vi "Read (Digital Waveform).vi"(8 "error in (no error)":errorcluster, 9 "Timeout (10000 ms)":u32=10000, 11 "VISA resource name":refnum<visa-resource-name>) -> (0 "error out":errorcluster, 2 "Digital Waveform Graph":digitalwaveform(graph), 3 "VISA resource name out":refnum<visa-resource-name>)   [LabVIEW 2023, in "RIGOL DS1054Z.lvlib"]
doc: "Initiates an acquisition on all digital channels. The VI waits for the acquisition to complete and returns the waveform. If the oscilloscope did not complete the acquisition within the time period you specify with the <B>Timeout</B> control, the VI returns a timeout error. A common cause for a timeout error is the acquisition was not triggered. For example, the trigger level is out of range of the waveform.\n\n<b>Notes:</b>\n(1) This VI is only for DS1000D Series.\n(2) Please make sure turn on the Logic Analyzer using Switch Logic Analyzer State.vi before running this VI.\n(3)The unit of X-Axis is \"s\" only when the instrument is in running mode."
uses:
  RIGOL DS1054Z.lvlib
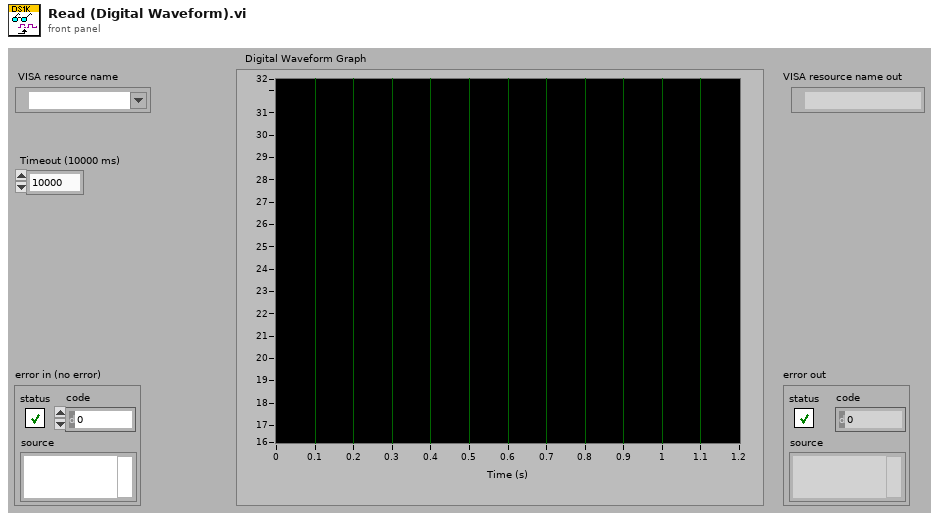
[diagram p1: front panel]
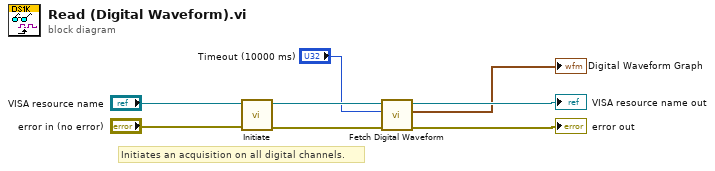
[diagram p0: block diagram]
diagram:
  # "Initiates an acquisition on all digital channels."
  n1 = call "Initiate.vi"("error in (no error)"="error in (no error)", "VISA resource name"="VISA resource name") -> ("error out"=w5:errorcluster, "VISA resource name out"=w6:refnum<visa-resource-name>)  [unwired: 8 out]
  n2 = call "Fetch Digital Waveform.vi"("error in (no error)"=w5, "Timeout (10000 ms)"="Timeout (10000 ms)", "VISA resource name"=w6) -> ("error out"=→"error out":errorcluster, "Digital Waveform Graph"=→"Digital Waveform Graph":digitalwaveform, "VISA resource name out"=→"VISA resource name out":refnum<visa-resource-name>)  [unwired: 6 out]
